vi "Write Pulse Delay.vi"(8 "error in":errorcluster, 10 "Delay":dbl, 11 "3300 in":refnum<class "3300.lvclass">) -> (0 "error out":errorcluster, 3 "3300 out":refnum<class "3300.lvclass">)   [LabVIEW 2019, in "3300.lvlib" / "3300.lvclass"]
uses:
  Library/3300.lvclass
  C:/Users/Public/Documents/Development/builds/Engine/Monitored Actor.lvlibp/Monitored Actor/Monitored Actor/Monitored Actor.lvclass
  builds/Engine/Monitored Actor.lvlibp/Monitored Actor/Monitored Actor/Read Actor Label.vi
  builds/Instruments/Electronic Load.lvlibp/Library/Electronic Load.lvclass
  builds/Instruments/Instruments.lvlibp/Library/Instruments.lvclass
  builds/Engine/Engine.lvlibp/Project/Engine.lvclass
  C:/Users/Public/Documents/Development/builds/Engine/Engine.lvlibp/Project/Engine.lvclass
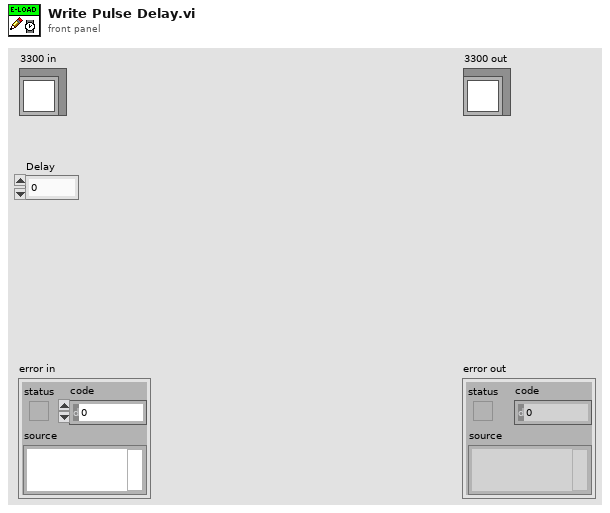
[diagram p1: front panel]
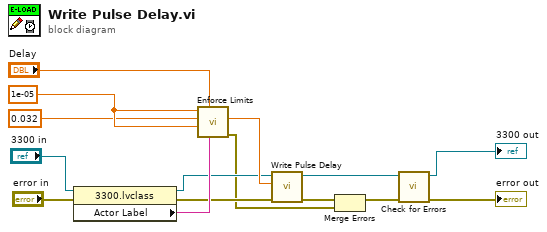
[diagram p0: block diagram]
diagram:
  w14 = 1e-05 ("lower limit")
  n1 = property class="3300.lvclass"(reference="3300 in", error in="error in") -> (reference out=w8:refnum<class "3300.lvclass">, error out=w7:errorcluster, "Actor Label"=w10:string)
  n2 = call "Enforce Limits.vi"("Device"=w10, "Setpoint"="Delay", "Minimum"=w14, "Maximum"=0.032 ("upper limit"), "Previous"=w14) -> ("error out"=w1:errorcluster, "Protected Setpoint"=w9:dbl)  [unwired: 5 in]
  n3 = call-parent "Write Pulse Delay.vi"("error in"=w7, "Delay"=w9, "Electronic Load in"=w8) -> ("error out"=w3:errorcluster, "Electronic Load out"=w6:refnum<class "3300.lvclass">)  [unwired: 7 in]
  n4 = Merge Errors(w3, w1) -> (w2:errorcluster)
  n5 = call "Check for Errors.vi"("error in"=w2, "Engine in"=w6) -> ("error out"=→"error out":errorcluster, "Engine out"=→"3300 out":refnum<class "3300.lvclass">)  [unwired: 8 in]
